vi "ReadHomeVoltage.vi"(11 "Handle":u32) -> (2 "At home":bool, 3 "Voltage read 0V=in position":dbl)   [LabVIEW 2020]
uses:
  cDaqlib/cDaq.lvlib
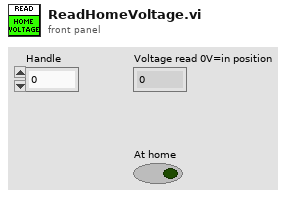
[diagram p1: front panel]
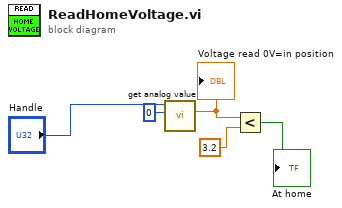
[diagram p0: block diagram]
diagram:
  n1 = call "get analog value .vi"("pin"=0, "daq"="Handle") -> ("function return"=w2:dbl)  [unwired: 8 in, 1 out]
  "Voltage read 0V=in position" <- w2
  n2 = Less?(x=w2, y=3.2) -> (x < y?=→"At home":bool)
